vi "Modify INI File.vi"(8 "error in (no error)":errorcluster, 11 "files generated by build":path[](array[path])) -> (0 "error out":errorcluster)   [LabVIEW 2025, in "I2C Bus Monitor.lvclass"]
uses:
  I2C Bus Monitor.lvclass
  I2C Bus Monitor.lvclass/I2C Bus Monitor.ctl
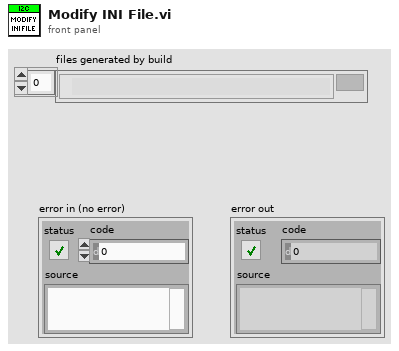
[diagram p1: front panel]
types:
  T1 = enum16{"open", "replace", "create", "open or create", "replace or create", "replace or create with confirmation"}
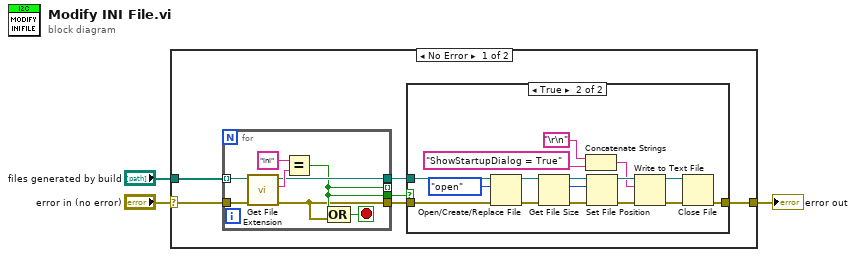
[diagram p0: block diagram]
diagram:
  n1 = case shown="No Error" "error in (no error)" {
    selector: "error in (no error)" -> [w8 w35]
    tunnel: [w9 w35] -> w3
    tunnel: "files generated by build" -> [w7 _]
    frame No Error {
      n2 = for {
        tunnel: w8 -> [w17]
        tunnel: w7 -> [w16] mode=indexing
        tunnel: [w12] -> w6 if=w11
        tunnel: [w11] -> _ mode=indexing
        tunnel: [w11] -> w4
        tunnel: [w10] -> w5
        stop <- w13 stop-if-true
        n3 = call <vilib>:"Get File Extension.vi"("error in (no error)"=w17, "file"=w16) -> ("error out"=w10:errorcluster, "lowercase file extension"=w15:string, "dup file"=w12:path)  [unwired: 5 in, 2 out]
        n4 = Equal?(x="ini", y=w15) -> (x = y?=w11:bool)
        n5 = Compound Arithmetic op=OR(w11, w10) -> (w13:bool)
      }
      n6 = case shown="True" w4 {
        tunnel: w5 -> [w18 w32]
        tunnel: [w18 w28] -> w9
        tunnel: w6 -> [_ w27]
        frame False {
        }
        frame True {
          n7 = Open/Create/Replace File(file path (use dialog)=w27, error in=w32, operation (0:open)=T1."open") -> (refnum out=w25:refnum<file>, error out=w33:errorcluster)  [unwired: 3 in, 1 out]
          n8 = Get File Size(file=w25, error in=w33) -> (refnum out=w23:refnum<file>, size (in bytes)=w21:i64, 0:w26:errorcluster)
          n9 = Concatenate Strings("\r\n", "ShowStartupDialog = True" ("text")) -> (w20:string)
          n10 = Set File Position(offset (in bytes) (0)=w21, refnum=w23, error in=w26) -> (refnum out=w22:refnum<file>, error out=w24:errorcluster)  [unwired: 1 in]
          n11 = Write to Text File(file (use dialog)=w22, text=w20, error in=w24) -> (refnum out=w29:refnum<file>, error out=w30:errorcluster)  [unwired: 1 in, 1 out]
          n12 = Close File(refnum=w29, error in=w30) -> (error out=w28:errorcluster)  [unwired: 1 out]
        }
      }
    }
    frame Error {
    }
  }
  "error out" <- w3
